vi "Destroy.vi"(0 "reference":refnum<class "ClassRelationshipEdge.lvclass">, 5 "error in (no error)":errorcluster) -> (19 "error out":errorcluster)   [LabVIEW 2014, in "ClassRelationshipEdge.lvclass"]
doc: "Destroys a ClassRelationshipEdge object created with a ClassRelationshipEdge constructor VI.\n\n[GOOP 2.1]"
uses:
  <resource>/Framework/Providers/Open_GDS/UML/ClassRelationshipEdge_class/ClassRelationshipEdge.lvclass
  <resource>/Framework/Providers/Open_GDS/UML/SegmentedLineEdge_class/SegmentedLineEdge.lvclass
panel:
  out "reference out":refnum<class "ClassRelationshipEdge.lvclass">
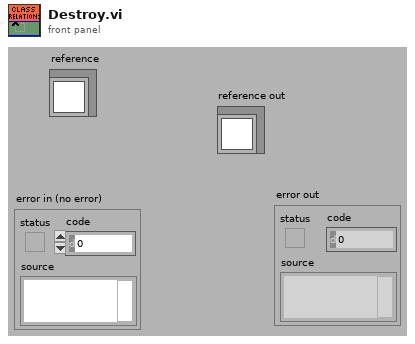
[diagram p1: front panel]
types:
  T1 = typedef "ClassRelationshipEdge.lvclass/ObjectAttributes.ctl" = cluster{"bentStyleRef":refnum<class "BentStyle.lvclass">, "startConnectionOffset":cluster{"x":i32, "y":i32}, "endConnectionOffset":cluster{"x":i32, "y":i32}, "MidLineOffset":cluster{"x":i32, "y":i32}, "DepClass":T2}
  T2 = typedef "ReversedEngineering_ViDependencyDetailsType.ctl" = cluster{"ThisVIs/Ctls":path[], "Dependent_VIs/Ctls":path[]}
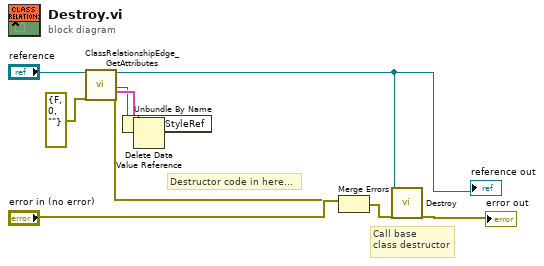
[diagram p0: block diagram]
diagram:
  # "Call base\nclass destructor"
  # "Destructor code in here..."
  n1 = call <resource>:"ClassRelationshipEdge_GetAttributes.vi"("reference in"="reference", "error in (no error)"=errorcluster {"status"=FALSE, "code"=0, "source"=""}) -> ("reference out"=w4:refnum<class "ClassRelationshipEdge.lvclass">, "Data"=w2:T1, "DataRef"=w1:refnum<data-value>, "error out"=w5:errorcluster)  [unwired: 1 in, 13 out]
  "reference out" <- w4
  n2 = Unbundle By Name(w2) -> ()  [unwired: 1 out]
  n3 = Delete Data Value Reference(data value reference=w1) -> ()  [unwired: 1 in, 2 out]
  n4 = Merge Errors("error in (no error)", w5) -> (w3:errorcluster)
  n5 = call-parent "Destroy.vi"("reference"=w4, "error in (no error)"=w3) -> ("error out"=→"error out":errorcluster)  [unwired: 17 in]
